vi "Register HTTP.vi"(8 "error in (no error)":errorcluster, 11 "Volatus Core in":refnum<class "Volatus Core.lvclass">) -> (0 "error out":errorcluster, 3 "Volatus Core out":refnum<class "Volatus Core.lvclass">)   [LabVIEW 2020, in "Volatus.lvlib" / "Volatus Core.lvclass"]
uses:
  Volatus Core.lvclass
  Volatus Core.lvclass/Volatus Core.ctl
  Module/Module.lvclass
  VolatusAPI/VolatusAPI.lvclass
  Config Type.ctl
  HomeHTTPController/HomeHTTPController.lvclass
  DebugHTTPController/DebugHTTPController.lvclass
  VolatusConfig/Node/Node Config.lvclass
  lv-vecto/Vecto/Node Config/Node Config.lvclass
  C:/dev/lv20CE/relink/lv-volatus/Volatus/Module/Module.lvclass
  C:/dev/lv20CE/relink/lv-volatus/Volatus/Volatus Core/Volatus Core.lvclass
  HTTP Manager/HTTP Manager.lvclass
  VolatusApiHttpService/VolatusApiHttpService.lvclass
  C:/dev/lv20CE/relink/lv-volatus/Volatus/VolatusApiHttpService/VolatusApiHttpService.lvclass
  C:/dev/lv20CE/relink/lv-http-server/HTTP Server/Service/Service.lvclass
  C:/dev/lv20CE/relink/lv-http-server/HTTP Server/Controller/Controller.lvclass
  C:/dev/lv20CE/relink/lv-http-server/HTTP Server/Handler/Handler.lvclass
  C:/dev/lv20CE/relink/lv-volatus/Volatus/HomeHTTPController/HomeHTTPController.lvclass
  C:/dev/lv20CE/relink/lv-volatus/Volatus/DebugHTTPController/DebugHTTPController.lvclass
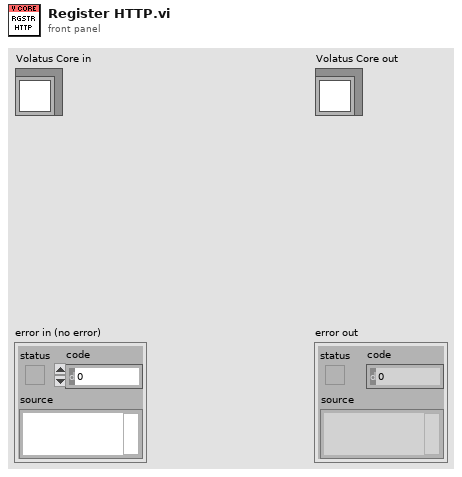
[diagram p1: front panel]
types:
  T1 = typedef "Volatus.lvlib/Volatus Core.lvclass/Config Type.ctl" = enum16{"App INI", "Memory", "Unconfigured"}
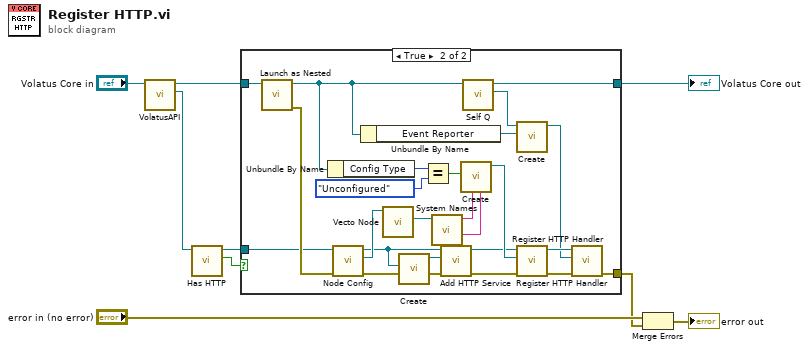
[diagram p0: block diagram]
diagram:
  n1 = call "VolatusAPI.vi"("Module in"="Volatus Core in") -> ("VolatusAPI"=w8:refnum<class "VolatusAPI.lvclass">, "Module out"=w5:refnum<class "Volatus Core.lvclass">)  [unwired: 9 in]
  n2 = call "Has HTTP.vi"("VolatusAPI in"=w8) -> ("Has HTTP"=w6:bool, "VolatusAPI out"=w4:refnum<class "VolatusAPI.lvclass">)  [unwired: 9 in]
  n3 = case shown="True" w6 {
    tunnel: w5 -> [w10 w28]
    tunnel: w4 -> [_ w22]
    tunnel: [w10 w17] -> w3
    tunnel: [_ w23] -> w1
    frame False {
    }
    frame True {
      n4 = call "Launch as Nested.vi"("Parent in"=w28) -> ("error out"=w33:errorcluster, "Parent"=w15:refnum<class "Volatus Core.lvclass">)  [unwired: 8 in, 1 out]
      n5 = Unbundle By Name(w15) -> ("Config Type"=w32:T1)
      n6 = call "Node Config.vi"("VolatusAPI in"=w22) -> ("Node Config"=w21:refnum<class "Node Config.lvclass">, "VolatusAPI out"=w11:refnum<class "VolatusAPI.lvclass">)  [unwired: 9 in]
      n7 = Unbundle By Name(w15) -> ("Event Reporter"=w27:refnum<class "MessageQ.lvclass">)
      n8 = call "Vecto Node.vi"("Node in"=w21) -> ("Vecto Node"=w20:refnum<class "Node Config.lvclass">)  [unwired: 8 in, 2 out]
      n9 = call "Create.vi"("VolatusAPI"=w11) -> ("VolatusApiHttpService out"=w12:refnum<class "VolatusApiHttpService.lvclass">)  [unwired: 10 in]
      n10 = Equal?(x=w32, y=Config_Type."Unconfigured") -> (x = y?=w30:bool)
      n11 = call "System Names.vi"("Node Config in"=w20) -> ("Name"=w18:string, "System"=w19:string)  [unwired: 8 in, 1 out]
      n12 = call "Add HTTP Service.vi"("error in (no error)"=w33, "Service"=w12, "VolatusAPI in"=w11) -> ("error out"=w14:errorcluster, "VolatusAPI out"=w13:refnum<class "VolatusAPI.lvclass">)  [unwired: 7 in]
      n13 = call "Create.vi"("Node"=w18, "System"=w19, "Unconfigured"=w30) -> ("HomeHTTPController out"=w29:refnum<class "HomeHTTPController.lvclass">)  [unwired: 7 in, 1 out]
      n14 = call "Self Q.vi"("Module in"=w15) -> ("Self Q"=w16:refnum<class "MessageQ.lvclass">, "Module out"=w17:refnum<class "Volatus Core.lvclass">)  [unwired: 9 in]
      n15 = call "Create.vi"("Event Module Q"=w27, "Core Module Q"=w16) -> ("DebugHTTPController out"=w24:refnum<class "DebugHTTPController.lvclass">)  [unwired: 8 in, 1 out]
      n16 = call "Register HTTP Handler.vi"("error in (no error)"=w14, "Handler"=w29, "VolatusAPI in"=w13) -> ("error out"=w26:errorcluster, "VolatusAPI out"=w25:refnum<class "VolatusAPI.lvclass">)  [unwired: 7 in]
      n17 = call "Register HTTP Handler.vi"("error in (no error)"=w26, "Handler"=w24, "VolatusAPI in"=w25) -> ("error out"=w23:errorcluster)  [unwired: 7 in, 1 out]
    }
  }
  "Volatus Core out" <- w3
  n18 = Merge Errors("error in (no error)", w1) -> (→"error out":errorcluster)
